vi "GetDrive.vi"   [LabVIEW 2020]
uses:
  DriveGlobals.vi
  <vilib>/Rock Robotics/Network Tables/NT Write Number.vi
types:
  T1 = typedef "WPI_EncoderDevRef.ctl" = cluster{"DevStatus":errorcluster, "EncoderIndex":T2, "CounterIndex":T3, "DistancePerCount":dbl, "Decoding Type":T4}
  T2 = typedef "FPGA_EncoderIdx.ctl" = enum8{"Enc 0", "Enc 1", "Enc 2", "Enc 3", "Enc 4", "Enc 5", "Enc 6", "Enc 7", "Invalid"}
  T3 = typedef "FPGA_CounterCtrSystemIndex.ctl" = enum8{"Ctr 0", "Ctr 1", "Ctr 2", "Ctr 3", "Ctr 4", "Ctr 5", "Ctr 6", "Ctr 7", "Invalid"}
  T4 = typedef "WPI_EncoderType.ctl" = enum16{"1x", "2x", "4x"}
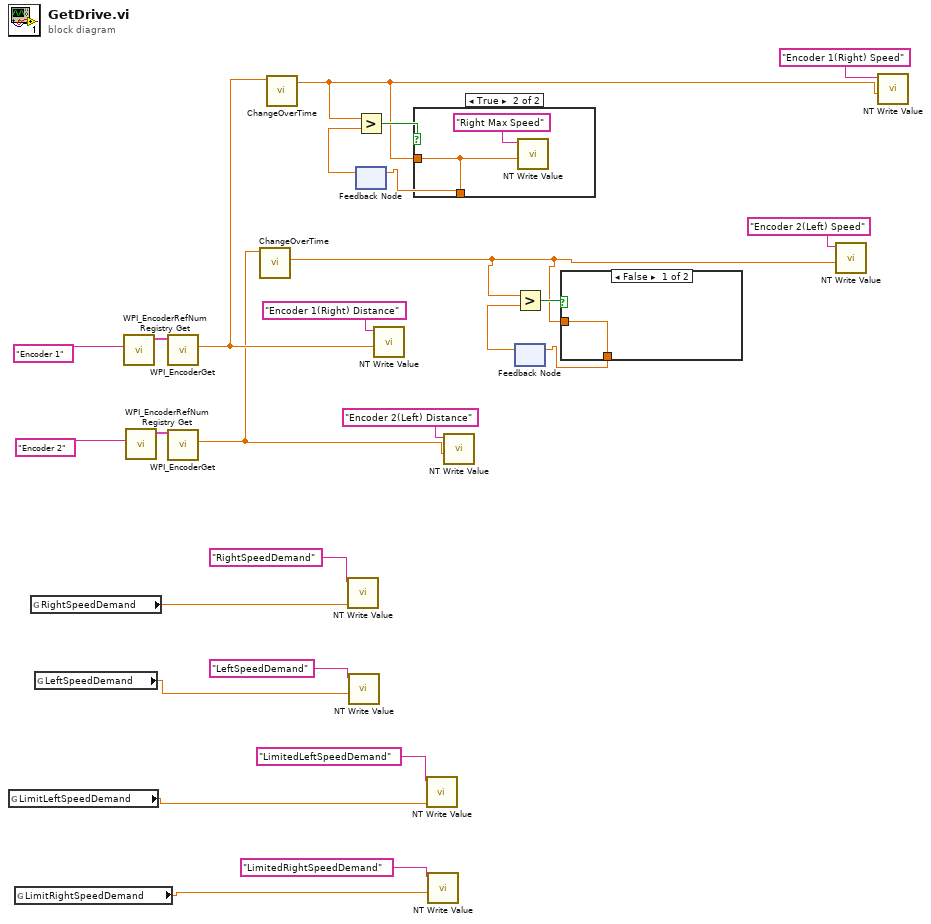
[diagram p0: block diagram]
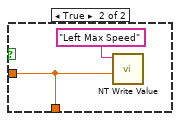
[diagram p2: hidden frame]
diagram:
  n1 = global read "DriveGlobals.vi" "LimitLeftSpeedDemand"() -> (w9:dbl)
  n2 = global read "DriveGlobals.vi" "LimitRightSpeedDemand"() -> (w10:dbl)
  n3 = global read "DriveGlobals.vi" "RightSpeedDemand"() -> (w16:dbl)
  n4 = global read "DriveGlobals.vi" "LeftSpeedDemand"() -> (w15:dbl)
  n5 = call <vilib>:"WPI_EncoderRefNum Registry Get.vi"("refnum name"="Encoder 1") -> ("EncoderDevRef"=w23:T1)  [unwired: 9 in, 1 out]
  n6 = call <vilib>:"WPI_EncoderRefNum Registry Get.vi"("refnum name"="Encoder 2") -> ("EncoderDevRef"=w24:T1)  [unwired: 9 in, 1 out]
  n7 = call <vilib>:"WPI_EncoderGet.vi"("EncoderDevRef"=w23) -> ("Distance"=w18:dbl)  [unwired: 5 in, 5 out]
  n8 = call <vilib>:"WPI_EncoderGet.vi"("EncoderDevRef"=w24) -> ("Distance"=w17:dbl)  [unwired: 5 in, 5 out]
  n9 = call "ChangeOverTime.vi"("InputNum"=w17) -> ("ChangeOverTime"=w1:dbl)  [unwired: 10 in]
  n10 = call "ChangeOverTime.vi"("InputNum"=w18) -> ("ChangeOverTime"=w7:dbl)  [unwired: 10 in]
  n11 = call-poly <vilib>:"NT Write Value.vi"("Numeric"=w16, "Name"="RightSpeedDemand") -> ()  [unwired: 9 in, 1 out]
  n12 = call-poly <vilib>:"NT Write Value.vi"("Numeric"=w15, "Name"="LeftSpeedDemand") -> ()  [unwired: 9 in, 1 out]
  n13 = feedback #1() -> (w5:dbl)  [unwired: 1 in]
  n14 = Greater?(x=w7, y=w5) -> (0:w8:bool)
  n15 = call-poly <vilib>:"NT Write Value.vi"("Numeric"=w18, "Name"="Encoder 1(Right) Distance") -> ()  [unwired: 9 in, 1 out]
  n16 = case shown="True" w8 {
    tunnel: w7 -> [w27 w28]
    tunnel: [w27 w28] -> w6
    frame False {
    }
    frame True {
      n17 = call-poly <vilib>:"NT Write Value.vi"("Numeric"=w28, "Name"="Right Max Speed") -> ()  [unwired: 9 in, 1 out]
    }
  }
  n18 = feedback-in #1(w6) -> ()
  n19 = call-poly <vilib>:"NT Write Value.vi"("Numeric"=w9, "Name"="LimitedLeftSpeedDemand") -> ()  [unwired: 9 in, 1 out]
  n20 = call-poly <vilib>:"NT Write Value.vi"("Numeric"=w10, "Name"="LimitedRightSpeedDemand") -> ()  [unwired: 9 in, 1 out]
  n21 = call-poly <vilib>:"NT Write Value.vi"("Numeric"=w17, "Name"="Encoder 2(Left) Distance") -> ()  [unwired: 9 in, 1 out]
  n22 = feedback #2() -> (w2:dbl)  [unwired: 1 in]
  n23 = Greater?(x=w1, y=w2) -> (0:w4:bool)
  n24 = case shown="False" w4 {
    tunnel: w1 -> [w30 w31]
    tunnel: [w30 w31] -> w3
    frame False {
    }
    frame True {
      n25 = call-poly <vilib>:"NT Write Value.vi"("Numeric"=w31, "Name"="Left Max Speed") -> ()  [unwired: 9 in, 1 out]
    }
  }
  n26 = feedback-in #2(w3) -> ()
  n27 = call-poly <vilib>:"NT Write Value.vi"("Numeric"=w1, "Name"="Encoder 2(Left) Speed") -> ()  [unwired: 9 in, 1 out]
  n28 = call-poly <vilib>:"NT Write Value.vi"("Numeric"=w7, "Name"="Encoder 1(Right) Speed") -> ()  [unwired: 9 in, 1 out]
